vi "force_priveliges_single_file.vi"(8 "error in (no error)":errorcluster, 11 "File path":path) -> (0 "error out":errorcluster, 3 "File path out":path)   [LabVIEW 2013]
panel:
  in  "Temp file folder":path=path "C:/Users/Clavius/Desktop"
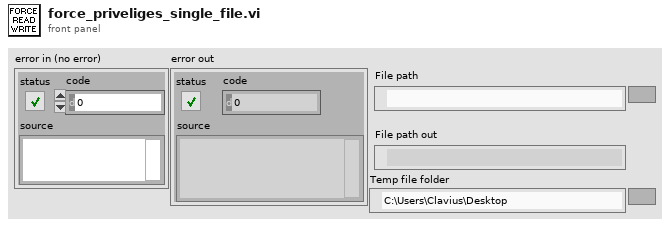
[diagram p1: front panel]
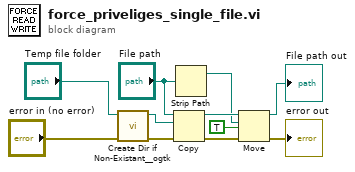
[diagram p0: block diagram]
diagram:
  n1 = call <userlib>:"Create Dir if Non-Existant__ogtk.vi"("error in (no error)"="error in (no error)", "Directory Path"="Temp file folder") -> ("error out"=w5:errorcluster, "dup Directory Path"=w4:path)  [unwired: 7 in, 1 out]
  n2 = Copy(8:w5, 10:w4, 11:"File path") -> (0:w8:errorcluster, 3:w7:path)  [unwired: 2 in, 1 out]
  n3 = Strip Path(path="File path") -> (stripped path=w2:path)  [unwired: 1 out]
  n4 = Move(source path=w7, error in=w8, 9:TRUE ("overwrite (F)"), 10:w2) -> (error out=→"error out":errorcluster, 3:→"File path out":path)  [unwired: 1 in, 1 out]
